vi "Send.vi"(8 "error in (no error)":errorcluster, 11 "Response in":refnum<class "Response.lvclass">) -> (0 "error out":errorcluster)   [LabVIEW 2023, in "Response.lvclass"]
uses:
  Response.lvclass
  <vilib>/Utility/error.llb/DialogType.ctl
  Response.lvclass/Response.ctl
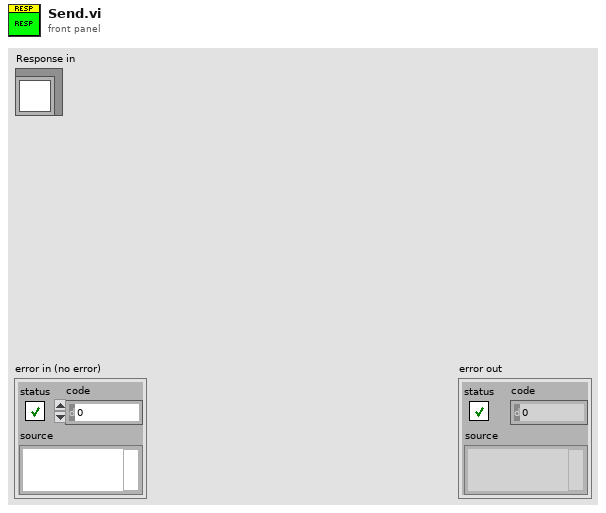
[diagram p1: front panel]
types:
  T1 = typedef "DialogType.ctl" = u16
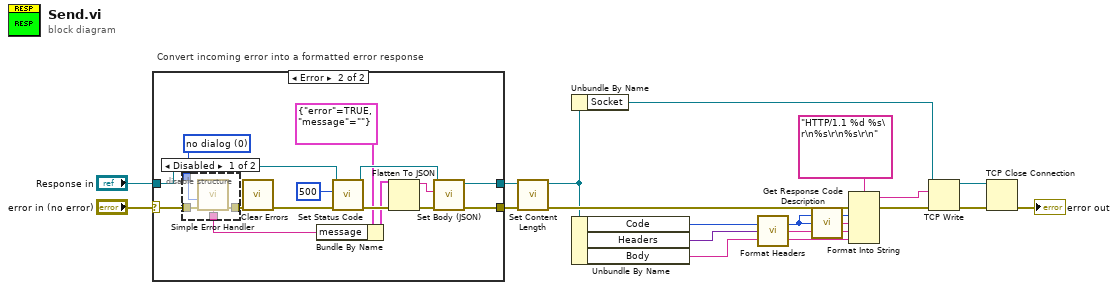
[diagram p0: block diagram]
diagram:
  # "Convert incoming error into a formatted error response"
  n1 = case shown="Error" "error in (no error)" {
    selector: "error in (no error)" -> [w19 w24]
    tunnel: "Response in" -> [w20 w23]
    tunnel: [w19 w22] -> w2
    tunnel: [w20 w21] -> w1
    frame No Error {
    }
    frame Error {
      w25 = T1 0 items=["no dialog", "OK message", "continue or stop message", "OK message + warnings", "continue/stop + warnings"] ("type of dialog (OK msg:1)")
      n2 = disable-structure shown="Disabled" {
        disable-tunnel: [w39 _] -> w30
        disable-tunnel: [w38 _] -> w26
        disable-tunnel: w25 -> [w37 _]
        disable-tunnel: w24 -> [w36 _]
        frame Disabled {
          n3 = call <vilib>:"Simple Error Handler.vi"("type of dialog (OK msg:1)"=w37, "error in (no error)"=w36) -> ("error out"=w39:errorcluster, "message"=w38:string)  [unwired: 3 in, 3 out]
        }
        frame Enabled {
        }
      }
      n4 = call <vilib>:"Clear Errors.vi"("error in (no error)"=w30) -> ("error out"=w29:errorcluster)  [unwired: 5 in, 1 out]
      n5 = Bundle By Name(cluster=cluster{"error":bool, "message":string} {"error"=TRUE, "message"=""}, "message"=w26) -> (w27:cluster{"error":bool, "message":string})
      n6 = call "Set Status Code.vi"("error in (no error)"=w29, "Status Code"=u16 500, "Response in"=w23) -> ("error out"=w35:errorcluster, "Response out"=w32:refnum<class "Response.lvclass">)  [unwired: 7 in]
      n7 = Flatten To JSON(anything=w27, error in (no error)=w35) -> (JSON string=w31:string, 11:w33:errorcluster)  [unwired: 1 in]
      n8 = call "Set Body (JSON).vi"("error in (no error)"=w33, "Body (as JSON)"=w31, "Response in"=w32) -> ("error out"=w22:errorcluster, "Response out"=w21:refnum<class "Response.lvclass">)  [unwired: 7 in]
    }
  }
  n9 = call "Set Content Length.vi"("error in (no error)"=w2, "Response in"=w1) -> ("error out"=w14:errorcluster, "Response out"=w7:refnum<class "Response.lvclass">)  [unwired: 8 in]
  n10 = Unbundle By Name(w7) -> ("Socket"=w6:refnum<k5>)
  n11 = Unbundle By Name(w7) -> ("Code"=w15:u16, "Headers"=w12:variant, "Body"=w11:string)
  n12 = call "Format Headers.vi"("Headers"=w12) -> ("Headers"=w13:string)
  n13 = call "Get Response Code Description.vi"("Code"=w15) -> ("Headers"=w16:string)
  n14 = Format Into String(format string="HTTP/1.1 %d %s\r\n%s\r\n%s\r\n", error in=w14, w15, w16, w13, w11) -> (resulting string=w9:string, error out=w17:errorcluster)  [unwired: 1 in]
  n15 = TCP Write(connection ID=w6, data in=w9, error in (no error)=w17) -> (connection ID out=w8:refnum<k5>, error out=w10:errorcluster)  [unwired: 1 in, 1 out]
  n16 = TCP Close Connection(connection ID=w8, error in (no error)=w10) -> (error out=→"error out":errorcluster)  [unwired: 1 in, 1 out]
